vi "odor config array property control (sub-vi).vi"(8 "error in (no error)":errorcluster, 9 "disable on error? (T)":bool=TRUE, 10 "re/initialize (F)":bool, 11 "odor config array refnum":refnum<vi>) -> (0 "error out":errorcluster, 3 "odor config array refnum out":refnum<vi>)   [LabVIEW 2021]
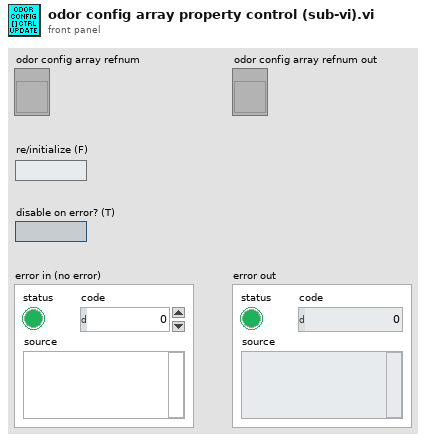
[diagram p1: front panel]
types:
  T1 = enum8{"Enabled", "Disabled", "Disabled and Grayed Out"}
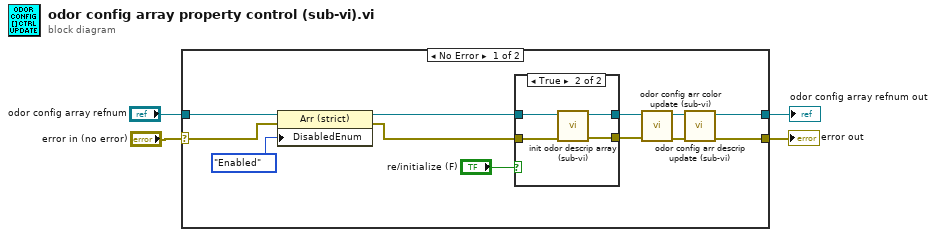
[diagram p0: block diagram]
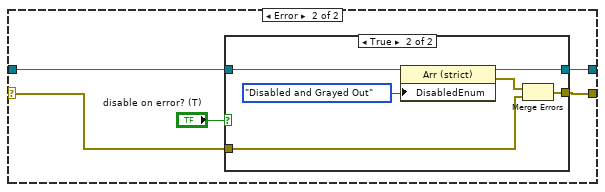
[diagram p3: hidden frame]
diagram:
  n1 = case shown="No Error" "error in (no error)" {
    selector: "error in (no error)" -> [w6 w25]
    tunnel: "odor config array refnum" -> [w8 w27]
    tunnel: [w15 w26] -> w2
    tunnel: [w14 w24] -> w1
    frame No Error {
      n2 = property class="Arr (strict)"(reference=w8, error in=w6, "DisabledEnum"=T1."Enabled" ("Disabled")) -> (reference out=w9:refnum<vi>, error out=w5:errorcluster)
      n3 = case shown="True" "re/initialize (F)" {
        tunnel: w9 -> [w18 w22]
        tunnel: w5 -> [w17 w20]
        tunnel: [w17 w19] -> w11
        tunnel: [w18 w21] -> w10
        frame False {
        }
        frame True {
          n4 = call "init odor descrip array (sub-vi).vi"("error in (no error)"=w20, "array refnum"=w22) -> ("error out"=w19:errorcluster, "array refnum out"=w21:refnum<vi>)  [unwired: 8 in]
        }
      }
      n5 = call "odor config arr color update (sub-vi).vi"("error in (no error)"=w11, "array refnum"=w10) -> ("error out"=w13:errorcluster, "array refnum out"=w12:refnum<vi>)  [unwired: 8 in]
      n6 = call "odor config arr descrip update (sub-vi).vi"("error in (no error)"=w13, "array refnum"=w12) -> ("error out"=w14:errorcluster, "array refnum out"=w15:refnum<vi>)  [unwired: 8 in]
    }
    frame Error {
      n7 = case shown="True" "disable on error? (T)" {
        tunnel: w27 -> [w28 w35]
        tunnel: [w28 w33] -> w26
        tunnel: w25 -> [w29 w31]
        tunnel: [w29 w30] -> w24
        frame False {
        }
        frame True {
          n8 = property class="Arr (strict)"(reference=w35, "DisabledEnum"=T1."Disabled and Grayed Out" ("Disabled")) -> (reference out=w33:refnum<vi>, error out=w32:errorcluster)  [unwired: 1 in]
          n9 = Merge Errors(w32, w31) -> (w30:errorcluster)
        }
      }
    }
  }
  "odor config array refnum out" <- w2
  "error out" <- w1
